vi "FRCts20_EspEngine_EspEngine.vi"(0 "httpRequestID":u32, 5 "Cluster":variant, 7 "Page":string, 9 "SearchBrowser":T1, 11 "error in (no error)":errorcluster) -> (4 "httpRequestID out":u32, 15 "error out":errorcluster)   [LabVIEW 2013, in "FRCts20_EspEngine.lvlib"]
uses:
  FRCts20_EspEngine.lvlib
  Backend/source/VI Source/FRCts20_Backend_API/FRCts20_Backend_API_Status.ctl
  Backend/source/VI Source/FRCts20_Backend_API/FRCts20_Backend_API.lvlib
  Backend/source/VI Source/FRCts20_Backend_API/FRCts20_Backend_API_SW.ctl
  <vilib>/wsapi/NI_WebServices.lvlib
  <vilib>/regexp/Match Regular Expression.xnode
  TypeDefs/FRCts20_EspEngine_Team.ctl
  TypeDefs/FRCts20_EspEngine_Event.ctl
  TypeDefs/FRCts20_EspEngine_Universe.ctl
  Web Methods/source/VI Source/Web Method Public Interface/FRCts20_WebMethods_ctl_request.ctl
  Web Methods/source/VI Source/FRCts20_WebMethods.lvlib
  Web Methods/source/VI Source/Web Method Public Interface/FRCts20_WebMethods_ctl_teamIdentifier.ctl
  Web Methods/source/VI Source/Web Method Public Interface/FRCts20_WebMethods_ctl_singleTeam.ctl
  Web Methods/source/VI Source/Web Method Public Interface/FRCts20_WebMethods_ctl_singleEvent.ctl
  TypeDefs/FRCts20_EspEngine_Request.ctl
  TypeDefs/FRCts20_EspEngine_AdvancedComponents_Bar.ctl
  TypeDefs/FRCts20_EspEngine_RequestPerHour_Line.ctl
  TypeDefs/FRCts20_EspEngine_SwUsage_Pie.ctl
  <vilib>/wsapi/subVIs/Set String ESP Variable.vi
  TypeDefs/FRCts20_EspEngine_SearchBrowser.ctl
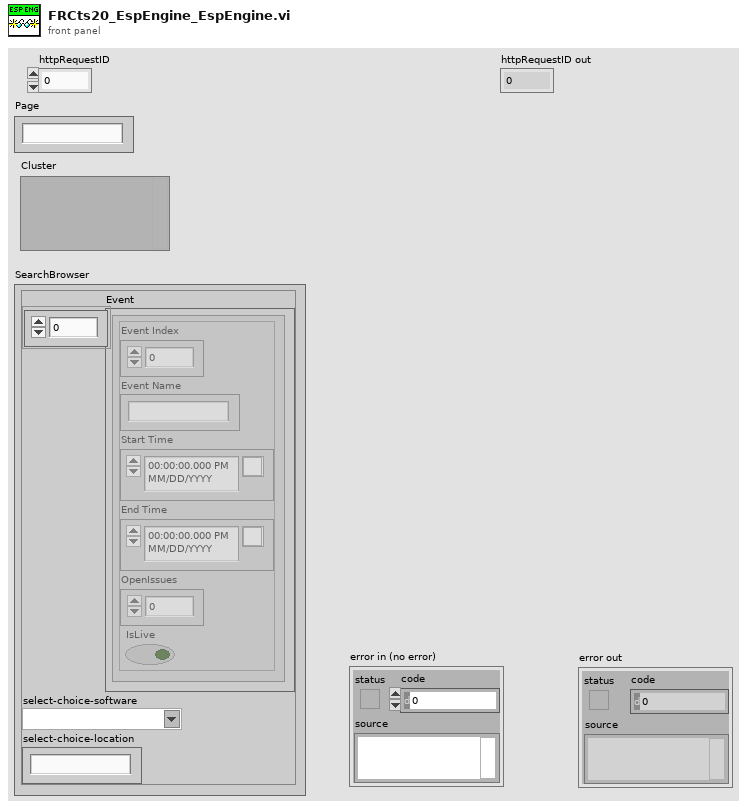
[diagram p1: front panel]
types:
  T1 = typedef "FRCts20_EspEngine.lvlib/FRCts20_EspEngine_SearchBrowser.ctl" = cluster{"Event":cluster{"Event Index":u32, "Event Name":string, "Start Time":timestamp, "End Time":timestamp, "OpenIssues":u8, "IsLive":bool}[], "select-choice-software":string, "select-choice-location":string}
  T2 = typedef "FRCts20_EspEngine.lvlib/FRCts20_EspEngine_Universe.ctl" = cluster{"TeamsListLength":i16, "Teams":T3[], "LiveEventListLength":i16, "LiveEvents":T9[], "NonLiveEventListLength":i16, "NonLiveEvents":T9[], "OpenIssueCount":i16, "NotFoundStatus":bool}
  T3 = typedef "FRCts20_EspEngine.lvlib/FRCts20_EspEngine_Team.ctl" = cluster{"Team":T4, "RequestListLength":i16, "Requests":T7[]}
  T4 = typedef "FRCts20_WebMethods.lvlib/FRCts20_WebMethods_ctl_singleTeam.ctl" = cluster{"Events":string[], "Robot Name":string, "Kinect":bool, "Vision":bool, "Can":bool, "Tags":string, "Avatar URL":string, "Team":T5, "SWType":T6}
  T5 = typedef "FRCts20_WebMethods.lvlib/FRCts20_WebMethods_ctl_teamIdentifier.ctl" = cluster{"Team Nickname":string, "Team Number ":u32, "UniqueId":u32}
  T6 = typedef "FRCts20_Backend_API.lvlib/FRCts20_Backend_API_SW.ctl" = string
  T7 = typedef "FRCts20_WebMethods.lvlib/FRCts20_WebMethods_ctl_request.ctl" = cluster{"Event":string, "Description":string, "Status":T8, "Open Date":string, "Last Update":string, "Close Date":string, "UniqueId":i32, "Team":cluster{"Team Nickname":string, "Team Number ":i32, "UniqueId":i32}, "Comments":cluster{"Request Number":dbl, "Text":string, "Author":string, "IsSolution":bool, "Team":cluster{"Team Nickname":string, "Team Identifier ":dbl}, "UniqueId":i32}[]}
  T8 = typedef "FRCts20_Backend_API.lvlib/FRCts20_Backend_API_Status.ctl" = enum16{"Open", "In Work", "Closed"}
  T9 = typedef "FRCts20_EspEngine.lvlib/FRCts20_EspEngine_Event.ctl" = cluster{"Single Event":T10, "EventOpenIssueCount":i16, "Requests":cluster{"RequestId":i32, "Request Description":string, "Team Number":i32}[], "ClosedRequests":cluster{"RequestId":i32, "Request Description":string, "Team Number":i32}[], "NotFoundStatus":bool}
  T10 = typedef "FRCts20_WebMethods.lvlib/FRCts20_WebMethods_ctl_singleEvent.ctl" = cluster{"Team":T5[], "Issue Count":i32, "Location":string, "Start Date ":timestamp}
  T11 = typedef "FRCts20_EspEngine.lvlib/FRCts20_EspEngine_Request.ctl" = cluster{"Request":T7, "CommentListLength":i16}
  T12 = typedef "FRCts20_EspEngine.lvlib/FRCts20_EspEngine_SwUsage_Pie.ctl" = cluster{"Live Event Location":string, "LabVIEW":dbl, "C++":dbl, "Java":dbl, "Other":dbl, "TotalTeams":i32, "TeamsReporting":i32}[]
  T13 = typedef "FRCts20_EspEngine.lvlib/FRCts20_EspEngine_RequestPerHour_Line.ctl" = cluster{"StartDate":cluster{"Year":i32, "Month":i32, "Day":i32}, "Events":cluster{"Location":string, "Requests":i32[]}[]}
  T14 = typedef "FRCts20_EspEngine.lvlib/FRCts20_EspEngine_AdvancedComponents_Bar.ctl" = cluster{"CAN":i32, "Vision":i32, "Kinect":i32}
  T15 = cluster{"SW Usage Pies":T12, "RequestsPerHour":T13, "Advanced Components":T14}
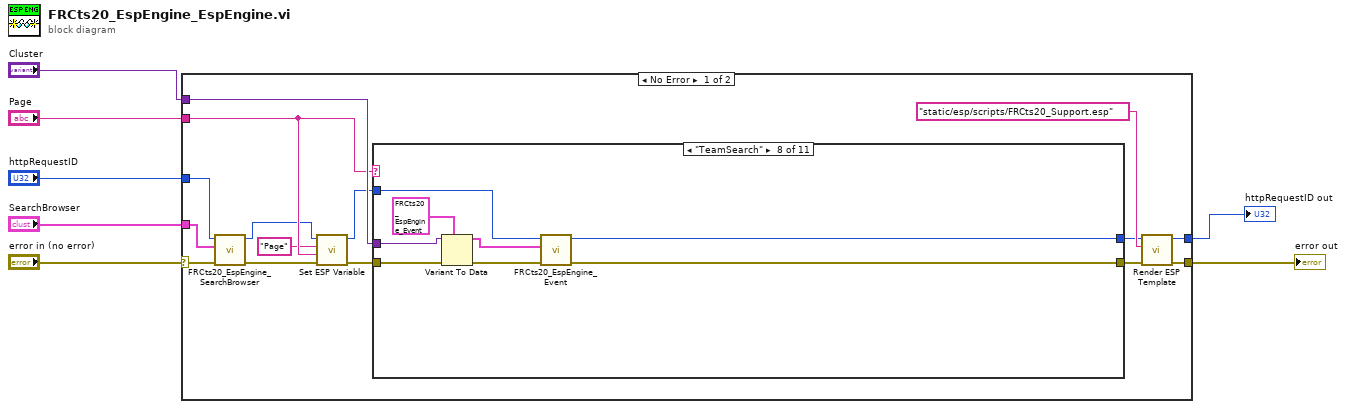
[diagram p0: block diagram]
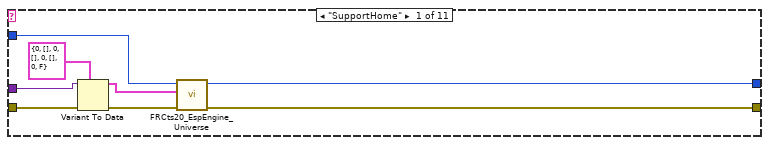
[diagram p2: hidden frame]
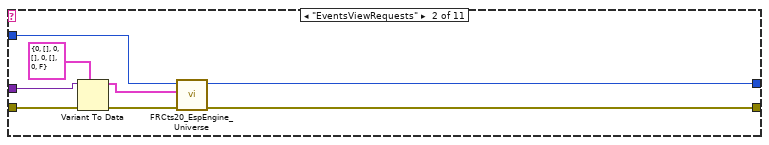
[diagram p3: hidden frame]
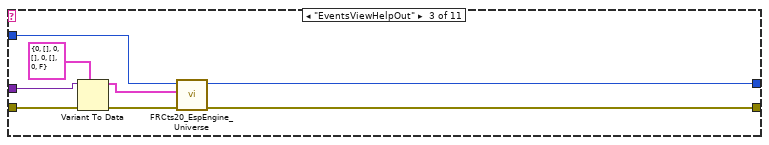
[diagram p4: hidden frame]
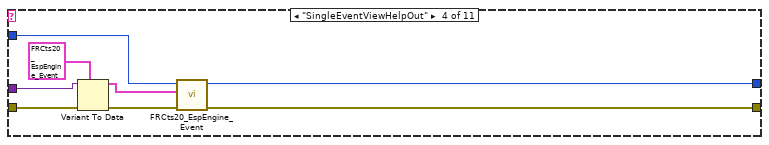
[diagram p5: hidden frame]
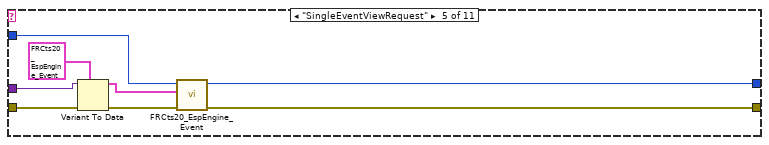
[diagram p6: hidden frame]
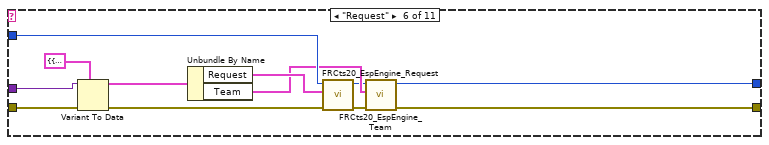
[diagram p7: hidden frame]
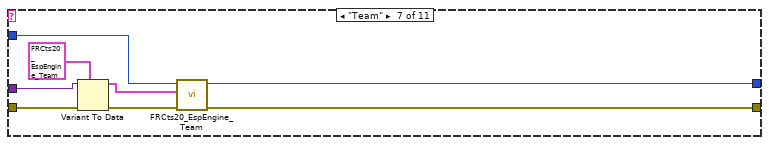
[diagram p8: hidden frame]
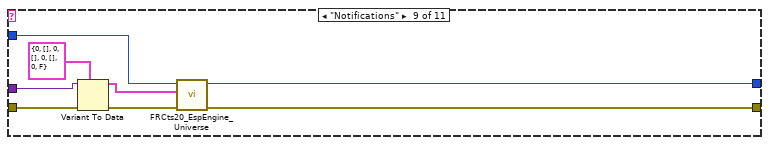
[diagram p9: hidden frame]
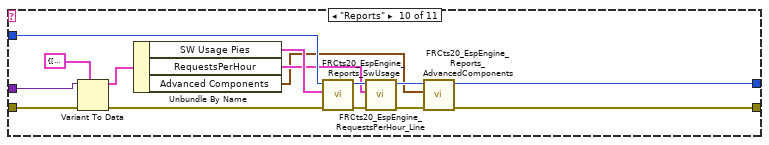
[diagram p10: hidden frame]
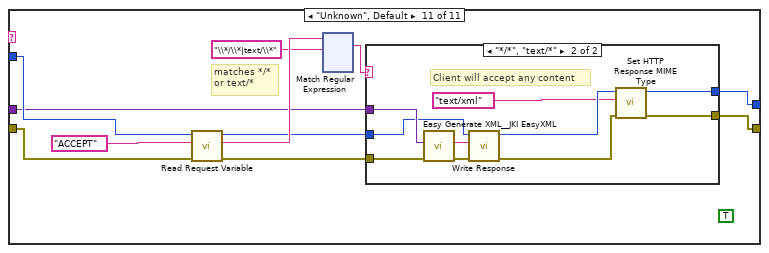
[diagram p11: hidden frame]
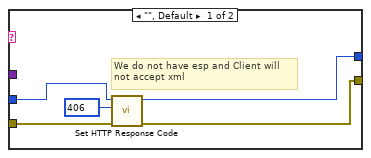
[diagram p12: hidden frame]
diagram:
  n1 = case shown="No Error" "error in (no error)" {
    selector: "error in (no error)" -> [w12 w251]
    tunnel: "Cluster" -> [w22 _]
    tunnel: "httpRequestID" -> [w10 w252]
    tunnel: [w18 w252] -> w5
    tunnel: [w19 w251] -> w3
    tunnel: "Page" -> [w14 _]
    tunnel: "SearchBrowser" -> [w11 _]
    frame No Error {
      n2 = call "FRCts20_EspEngine_SearchBrowser.vi"("error in (no error)"=w12, "SearchBrowser"=w11, "httpRequestID"=w10) -> ("error out"=w9:errorcluster, "httpRequestID out"=w8:u32)  [unwired: 7 in]
      n3 = call-poly <vilib>:"Set ESP Variable.vi"("error in (no error)"=w9, "value"=w14, "key"="Page", "httpRequestID"=w8) -> ("error out"=w20:errorcluster, "httpRequestID out"=w21:u32)  [unwired: 6 in]
      n4 = case shown="\"TeamSearch\"" w14 {
        tunnel: w22 -> [w29 w34 w39 w53 w58 w74 w82 w90 w94 w113 w116]
        tunnel: w21 -> [w27 w33 w41 w50 w59 w71 w79 w83 w95 w110 w124]
        tunnel: w20 -> [w28 w35 w40 w54 w57 w72 w78 w89 w93 w112 w122]
        tunnel: [w23 w32 w43 w47 w56 w65 w75 w85 w91 w100 w115] -> w16
        tunnel: [w24 w31 w42 w49 w55 w63 w77 w84 w92 w99 w114] -> w15
        frame "SupportHome" {
          n5 = Variant To Data(error in=w28, type=T2 {"TeamsListLength"=0, "Teams"=[], "LiveEventListLength"=0, "LiveEvents"=[], "NonLiveEventListLength"=0, "NonLiveEvents"=[], "OpenIssueCount"=0, "NotFoundStatus"=FALSE} ("Universe"), Variant=w29) -> (data=w26:T2, error out=w25:errorcluster)
          n6 = call "FRCts20_EspEngine_Universe.vi"("error in (no error)"=w25, "Universe"=w26, "httpRequestID"=w27) -> ("error out"=w23:errorcluster, "httpRequestID out"=w24:u32)  [unwired: 7 in]
        }
        frame "EventsViewRequests" {
          n7 = Variant To Data(error in=w35, type=T2 {"TeamsListLength"=0, "Teams"=[], "LiveEventListLength"=0, "LiveEvents"=[], "NonLiveEventListLength"=0, "NonLiveEvents"=[], "OpenIssueCount"=0, "NotFoundStatus"=FALSE} ("Universe"), Variant=w34) -> (data=w37:T2, error out=w38:errorcluster)
          n8 = call "FRCts20_EspEngine_Universe.vi"("error in (no error)"=w38, "Universe"=w37, "httpRequestID"=w33) -> ("error out"=w32:errorcluster, "httpRequestID out"=w31:u32)  [unwired: 7 in]
        }
        frame "EventsViewHelpOut" {
          n9 = Variant To Data(error in=w40, type=T2 {"TeamsListLength"=0, "Teams"=[], "LiveEventListLength"=0, "LiveEvents"=[], "NonLiveEventListLength"=0, "NonLiveEvents"=[], "OpenIssueCount"=0, "NotFoundStatus"=FALSE} ("Universe"), Variant=w39) -> (data=w45:T2, error out=w46:errorcluster)
          n10 = call "FRCts20_EspEngine_Universe.vi"("error in (no error)"=w46, "Universe"=w45, "httpRequestID"=w41) -> ("error out"=w43:errorcluster, "httpRequestID out"=w42:u32)  [unwired: 7 in]
        }
        frame "SingleEventViewHelpOut" {
          n11 = Variant To Data(error in=w54, type=T9 {"Single Event"={"Team"=[], "Issue Count"=0, "Location"="", "Start Date "=timestamp(0 s since 1904-01-01)}, "EventOpenIssueCount"=0, "Requests"=[], "ClosedRequests"=[], "NotFoundStatus"=FALSE} ("Event"), Variant=w53) -> (data=w51:T9, error out=w48:errorcluster)
          n12 = call "FRCts20_EspEngine_Event.vi"("error in (no error)"=w48, "Event"=w51, "httpRequestID"=w50) -> ("error out"=w47:errorcluster, "httpRequestID out"=w49:u32)  [unwired: 7 in]
        }
        frame "SingleEventViewRequest" {
          n13 = Variant To Data(error in=w57, type=T9 {"Single Event"={"Team"=[], "Issue Count"=0, "Location"="", "Start Date "=timestamp(0 s since 1904-01-01)}, "EventOpenIssueCount"=0, "Requests"=[], "ClosedRequests"=[], "NotFoundStatus"=FALSE} ("Event"), Variant=w58) -> (data=w61:T9, error out=w60:errorcluster)
          n14 = call "FRCts20_EspEngine_Event.vi"("error in (no error)"=w60, "Event"=w61, "httpRequestID"=w59) -> ("error out"=w56:errorcluster, "httpRequestID out"=w55:u32)  [unwired: 7 in]
        }
        frame "Request" {
          n15 = Variant To Data(error in=w72, type=cluster{"Request":T11, "Team":T3} {"Request"={"Request"={"Event"="", "Description"="", "Status"=enum."Open", "Open Date"="", "Last Update"="", "Close Date"="", "UniqueId"=0, "Team"={"Team Nickname"="", "Team Number "=0, "UniqueId"=0}, "Comments"=[]}, "CommentListLength"=0}, "Team"={"Team"={"Events"=[], "Robot Name"="", "Kinect"=FALSE, "Vision"=FALSE, "Can"=FALSE, "Tags"="", "Avatar URL"="", "Team"={"Team Nickname"="", "Team Number "=0, "UniqueId"=0}, "SWType"=""}, "RequestListLength"=0, "Requests"=[]}} ("output cluster"), Variant=w74) -> (data=w69:cluster{"Request":T11, "Team":T3}, error out=w73:errorcluster)
          n16 = Unbundle By Name(w69) -> ("Request"=w68:T11, "Team"=w67:T3)
          n17 = call "FRCts20_EspEngine_Request.vi"("error in (no error)"=w73, "Request"=w68, "httpRequestID"=w71) -> ("error out"=w66:errorcluster, "httpRequestID"=w64:u32)  [unwired: 7 in]
          n18 = call "FRCts20_EspEngine_Team.vi"("error in (no error)"=w66, "Team"=w67, "httpRequestID"=w64) -> ("error out"=w65:errorcluster, "httpRequestID out"=w63:u32)  [unwired: 7 in]
        }
        frame "Team" {
          n19 = Variant To Data(error in=w78, type=T3 {"Team"={"Events"=[], "Robot Name"="", "Kinect"=FALSE, "Vision"=FALSE, "Can"=FALSE, "Tags"="", "Avatar URL"="", "Team"={"Team Nickname"="", "Team Number "=0, "UniqueId"=0}, "SWType"=""}, "RequestListLength"=0, "Requests"=[]} ("Team"), Variant=w82) -> (data=w80:T3, error out=w76:errorcluster)
          n20 = call "FRCts20_EspEngine_Team.vi"("error in (no error)"=w76, "Team"=w80, "httpRequestID"=w79) -> ("error out"=w75:errorcluster, "httpRequestID out"=w77:u32)  [unwired: 7 in]
        }
        frame "TeamSearch" {
          n21 = Variant To Data(error in=w89, type=T9 {"Single Event"={"Team"=[], "Issue Count"=0, "Location"="", "Start Date "=timestamp(0 s since 1904-01-01)}, "EventOpenIssueCount"=0, "Requests"=[], "ClosedRequests"=[], "NotFoundStatus"=FALSE} ("Event"), Variant=w90) -> (data=w87:T9, error out=w86:errorcluster)
          n22 = call "FRCts20_EspEngine_Event.vi"("error in (no error)"=w86, "Event"=w87, "httpRequestID"=w83) -> ("error out"=w85:errorcluster, "httpRequestID out"=w84:u32)  [unwired: 7 in]
        }
        frame "Notifications" {
          n23 = Variant To Data(error in=w93, type=T2 {"TeamsListLength"=0, "Teams"=[], "LiveEventListLength"=0, "LiveEvents"=[], "NonLiveEventListLength"=0, "NonLiveEvents"=[], "OpenIssueCount"=0, "NotFoundStatus"=FALSE} ("Universe"), Variant=w94) -> (data=w97:T2, error out=w98:errorcluster)
          n24 = call "FRCts20_EspEngine_Universe.vi"("error in (no error)"=w98, "Universe"=w97, "httpRequestID"=w95) -> ("error out"=w91:errorcluster, "httpRequestID out"=w92:u32)  [unwired: 7 in]
        }
        frame "Reports" {
          n25 = Variant To Data(error in=w112, type=T15 {"SW Usage Pies"=[], "RequestsPerHour"={"StartDate"={"Year"=0, "Month"=0, "Day"=0}, "Events"=[]}, "Advanced Components"={"CAN"=0, "Vision"=0, "Kinect"=0}} ("output cluster"), Variant=w113) -> (data=w109:T15, error out=w111:errorcluster)
          n26 = Unbundle By Name(w109) -> ("SW Usage Pies"=w108:T12, "RequestsPerHour"=w105:T13, "Advanced Components"=w101:T14)
          n27 = call "FRCts20_EspEngine_Reports_SwUsage.vi"("error in (no error)"=w111, "Software Usage Pie"=w108, "httpRequestID"=w110) -> ("error out"=w107:errorcluster, "httpRequestID out"=w106:u32)  [unwired: 7 in]
          n28 = call "FRCts20_EspEngine_RequestsPerHour_Line.vi"("error in (no error)"=w107, "RequestsPerHour"=w105, "httpRequestID"=w106) -> ("error out"=w102:errorcluster, "httpRequestID out"=w103:u32)  [unwired: 7 in]
          n29 = call "FRCts20_EspEngine_Reports_AdvancedComponents.vi"("error in (no error)"=w102, "Advanced Components"=w101, "httpRequestID"=w103) -> ("error out"=w100:errorcluster, "httpRequestID out"=w99:u32)  [unwired: 7 in]
        }
        frame "Unknown", Default {
          (unwired) TRUE
          # "matches */*\nor text/*"
          n30 = call <vilib>:"Read Request Variable.vi"("error in (no error)"=w122, "variable name"="ACCEPT", "httpRequestID"=w124) -> ("error out"=w118:errorcluster, "value"=w121:string, "httpRequestID out"=w117:u32)  [unwired: 6 in]
          n31 = xnode "Match Regular Expression"("input string"=w121, "regular expression"="\\*/\\*|text/\\*") -> ("whole match"=w119:string)  [unwired: 4 in, 4 out]
          n32 = case shown="\"*/*\", \"text/*\"" w119 {
            tunnel: w118 -> [w128 w136]
            tunnel: w117 -> [w129 w135]
            tunnel: w116 -> [_ w139]
            tunnel: [w127 w134] -> w115
            tunnel: [w126 w133] -> w114
            frame "", Default {
              w125 = 406 items=["100"=100, "101"=101, "200"=200, "201"=201, "202"=202, "203"=203, "204"=204, "205"=205, "206"=206, "300"=300, "301"=301, "302"=302, "303"=303, "304"=304, "305"=305, "306"=306, "307"=307, "400"=400, "401"=401, "402"=402, "403"=403, "404"=404, "405"=405, "406"=406, "407"=407, "408"=408, "409"=409, "410"=410, "411"=411, "412"=412, "413"=413, "414"=414, "415"=415, "416"=416, "417"=417, "500"=500, "501"=501, "502"=502, "503"=503, "504"=504, "505"=505] ("response code (200)")
              # "We do not have esp and Client will\nnot accept xml"
              n33 = call <vilib>:"Set HTTP Response Code.vi"("error in (no error)"=w128, "response code (200)"=w125, "httpRequestID"=w129) -> ("error out"=w127:errorcluster, "httpRequestID out"=w126:u32)  [unwired: 7 in]
            }
            frame "*/*", "text/*" {
              # "Client will accept any content"
              n34 = call <vilib>:"Easy Generate XML__JKI EasyXML.vi"("error in (no error)"=w136, "LabVIEW Data"=w139) -> ("error out"=w138:errorcluster, "XML String"=w137:string)  [unwired: 8 in]
              n35 = call <vilib>:"Write Response.vi"("error in (no error)"=w138, "response string"=w137, "httpRequestID"=w135) -> ("error out"=w132:errorcluster, "httpRequestID out"=w131:u32)  [unwired: 7 in]
              n36 = call <vilib>:"Set HTTP Response MIME Type.vi"("error in (no error)"=w132, "MIME type (text/html)"="text/xml", "httpRequestID"=w131) -> ("error out"=w134:errorcluster, "httpRequestID out"=w133:u32)  [unwired: 7 in]
            }
          }
        }
      }
      n37 = call <vilib>:"Render ESP Template.vi"("error in (no error)"=w16, "espName"="static/esp/scripts/FRCts20_Support.esp", "httpRequestID"=w15) -> ("error out"=w19:errorcluster, "httpRequestID out"=w18:u32)  [unwired: 7 in]
    }
    frame Error {
    }
  }
  "httpRequestID out" <- w5
  "error out" <- w3
